vi "AB_Engine_InteropAssembly_Get_ProtoInfo.vi"(6 "2011CompatibilityMode":bool, 7 "Path":path, 8 "error in (no error)":errorcluster, 9 "destinations":refnum<class "AB_Destination.lvclass">[](array[class]), 11 "sourceItems":refnum<class "AB_Source.lvclass">[](array[class])) -> (0 "error out":errorcluster, 2 "ExportAssemblyLVClassinfo":T1[](array[typedef]), 3 "ExportAssemblyVIinfo":T3[](array[typedef]))   [LabVIEW 2020]
uses:
  <vilib>/AppBuilder/AB_Classes/Source/AB_Source.lvclass
  <vilib>/AppBuilder/AB_InteropAssembly_DistVI_Proto_Info.ctl
  <vilib>/AppBuilder/IOStatus.ctl
  <vilib>/AppBuilder/AB_Classes/Destination/AB_Destination.lvclass
  <vilib>/AppBuilder/AB_InteropAssembly_DistVI_Class_Info.ctl
  <vilib>/AppBuilder/AB_Classes/Source/ExportedAssemblyVI/AB_Source_Exported_Assembly_VI.lvclass
  <vilib>/Utility/lvfile.llb/NI_FileType.lvlib
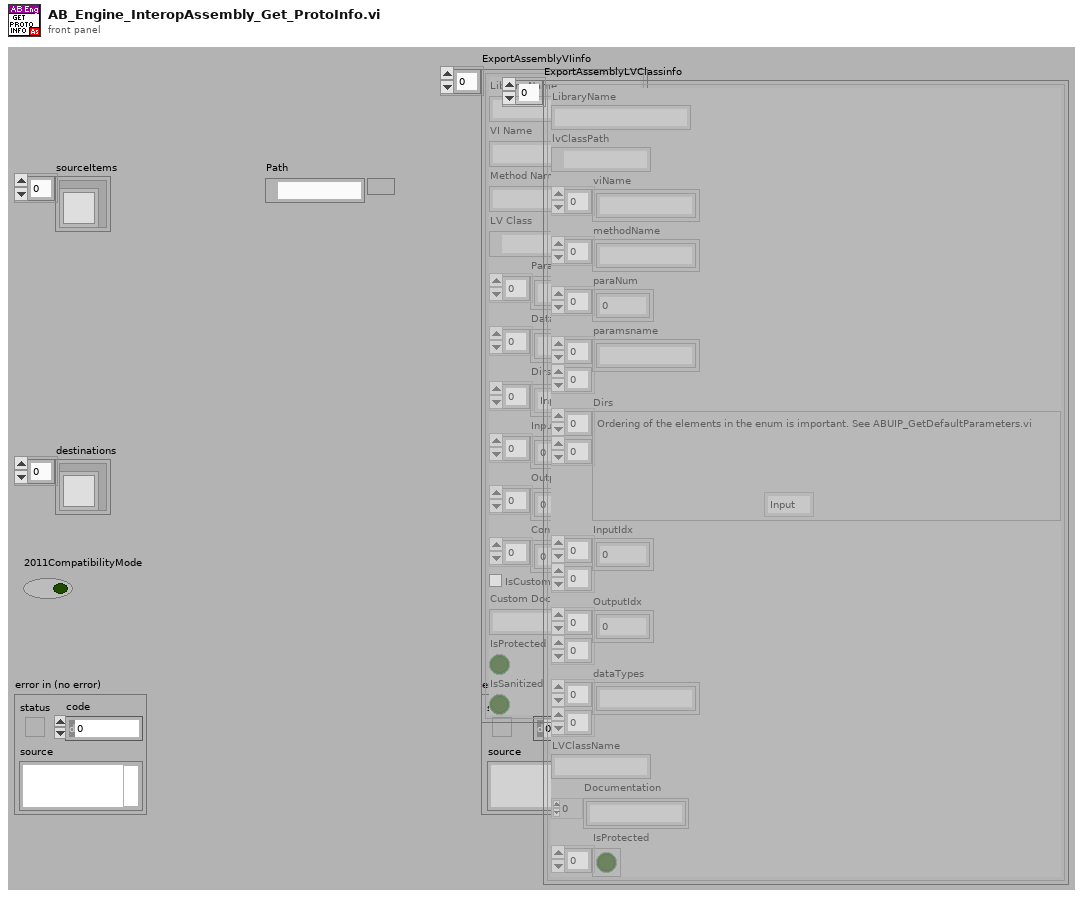
[diagram p1: front panel]
types:
  T1 = typedef "AB_InteropAssembly_DistVI_Class_Info.ctl" = cluster{"LibraryName":string, "lvClassPath":path, "viName":string[], "methodName":string[], "paraNum":i32[], "paramsname":string[][], "Dirs":T2[][], "InputIdx":i32[][], "OutputIdx":i32[][], "dataTypes":string[][], "LVClassName":string, "Documentation":string[], "IsProtected":bool[]}
  T2 = typedef "IOStatus.ctl" = enum16{"Input", "Output", "Input/Output", "InputDeleted", "OutputDeleted", "IODeleted", "ErrorClusterIn", "ErrorClusterOut"}
  T3 = typedef "AB_InteropAssembly_DistVI_Proto_Info.ctl" = cluster{"Library Name":string, "VI Name":string, "Method Name":string, "LV Class":path, "Param Names":string[], "Data Types":string[], "Dirs":T2[], "InputIdx":i32[], "OutputIdx":i32[], "ConNum":i8[], "IsCustomDocumentation":bool, "Custom Documentation":string, "IsProtected":bool, "IsSanitized":bool}
  T4 = cluster{"lvClassPath":path, "viName":string[], "methodName":string[], "paraNum":i32[], "paramsname":string[][], "Dirs":enum16{"in", "out", "in/out", "length"}[][], "InputIdx":i32[][], "OutputIdx":i32[][], "dataTypes":string[][], string}
  T5 = typedef "AB_Source.ctl" = cluster{"path":path, "itemID":string, "parentIndex":i32, "sourceInclusion":T6, "destinationIndex":i32, "properties":T7[], "newName":string, "lvfile":bool, "valid":bool, "eng_inBuild":bool, "eng_isNonVILink":bool, "Amalgamation":bool, "Amalgamation Piece":bool, "eng_delimitedName":string, "preventRename":bool}
  T6 = typedef "AB_Source_Inclusion.ctl" = enum16{"IncludeIfReferenced", "Include", "Exclude", "TopLevel"}
  T7 = typedef "AB_Source_Properties.ctl" = cluster{"sourcePropertyType":T8, "value":variant}
  T8 = typedef "AB_Source_Property_Type.ctl" = enum16{"Remove block diagram", "Remove front panel", "Password", "Window has title bar", "Show menu bar", "Show vertical scroll bar", "Show horizontal scroll bar", "Show toolbar", "Show Abort button", "Show fp when called", "Window behavior", "Allow user to close window", "Window run-time position", "Run when opened", "Allow debugging", "Auto error handling", "Generate guard code", "Use stack variables", "Expression folding", "Integer only", "Inline subVI"}
  T9 = typedef "AB_Destination.ctl" = cluster{"destName":string, "path":path, "libraryName":string, "preserveHierarchy":bool, "eng_inBuild":bool, "eng_libraryReference":refnum<vi>, "eng_restictAddToNewLibrary":bool}
  T10 = typedef "NI_FileType.lvlib/FT_FileTypes.ctl" = enum32{"Invalid file/path", "Unknown type", "Instrument", "Control", "Polymorphic VI", "Project", "Library", "LVClass", "XControl", "XNode", "CIN", "Run-time menu", "Palette menu", "LLB", "Shortcut", "Directory", "Class Private Data Control", "Statechart", "MathScript .m file", "Ladder Diagram", "LVLibp"}
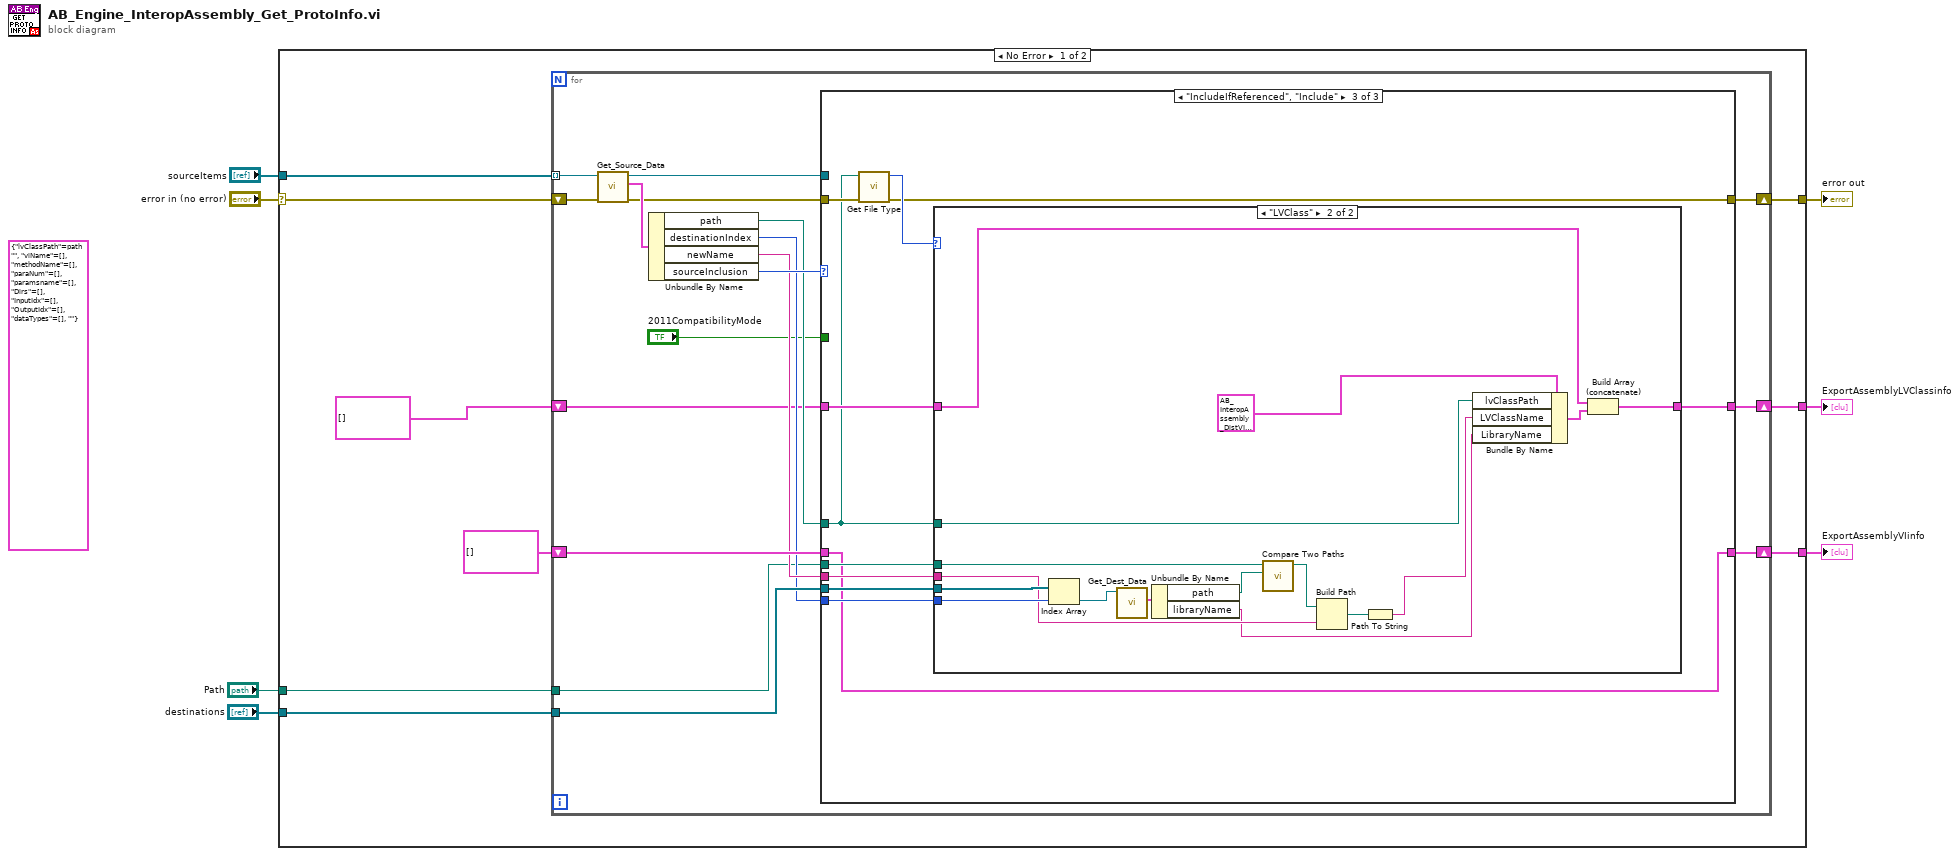
[diagram p0: block diagram]
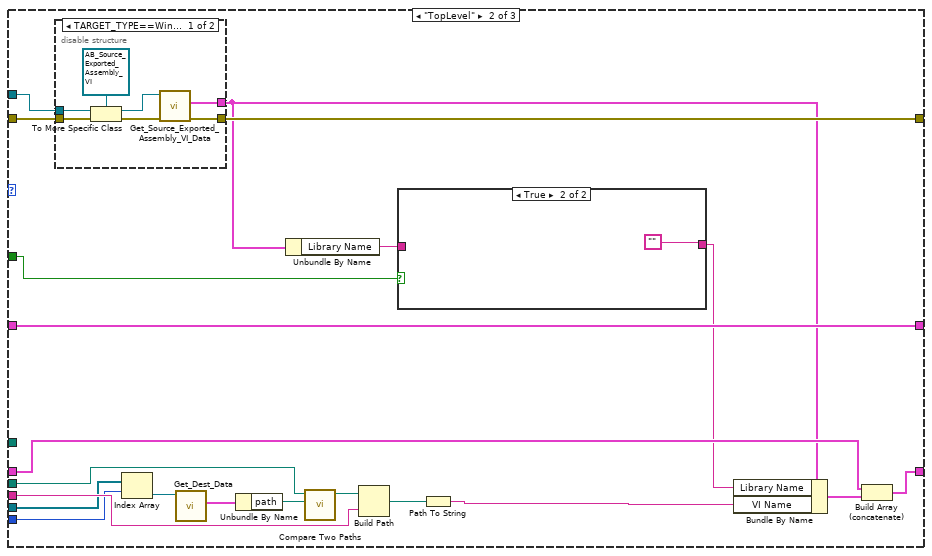
[diagram p3: hidden frame]
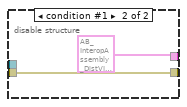
[diagram p5: hidden frame]
diagram:
  (unwired) T4 {"lvClassPath"=path "", "viName"=[], "methodName"=[], "paraNum"=[], "paramsname"=[], "Dirs"=[], "InputIdx"=[], "OutputIdx"=[], "dataTypes"=[], ""} ("ExportAssemblyVIinfo")
  n1 = case shown="No Error" "error in (no error)" {
    selector: "error in (no error)" -> [w15 w97]
    tunnel: "sourceItems" -> [w16 _]
    tunnel: [w14 _] -> w5
    tunnel: [w12 w97] -> w4
    tunnel: "destinations" -> [w11 _]
    tunnel: "Path" -> [w10 _]
    tunnel: [w8 _] -> w1
    frame No Error {
      n2 = for {
        tunnel: w16 -> [w32] mode=indexing
        shift-right: [w29] -> w12
        shift-left: w15 -> [w33]
        shift-right: [w31] -> w14
        shift-left: T3[] [] ("ExportAssemblyVIinfos") -> [w30]
        tunnel: w11 -> [w23]
        tunnel: w10 -> [w21]
        shift-right: [w18] -> w8
        shift-left: T1[] [] -> [w19]
        n3 = call <vilib>:"Get_Source_Data.vi"("error in (no error)"=w33, "Class in"=w32) -> ("error out"=w25:errorcluster, "data"=w28:T5, "Class out"=w26:refnum<class "AB_Source.lvclass">)  [unwired: 7 out]
        n4 = Unbundle By Name(w28) -> ("path"=w20:path, "destinationIndex"=w22:i32, "newName"=w24:string, "sourceInclusion"=w27:T6)
        n5 = case shown="\"IncludeIfReferenced\", \"Include\"" w27 {
          tunnel: w26 -> [_ w55 _]
          tunnel: w25 -> [w35 w54 w73]
          tunnel: [w36 w57 w74] -> w31
          tunnel: w30 -> [w36 w56 w74]
          tunnel: [w35 w53 w72] -> w29
          tunnel: w24 -> [_ w52 w77]
          tunnel: w23 -> [_ w49 w78]
          tunnel: w22 -> [_ w48 w79]
          tunnel: w21 -> [_ w47 w76]
          tunnel: w20 -> [_ _ w69]
          tunnel: w19 -> [w34 w46 w71]
          tunnel: [w34 w46 w70] -> w18
          tunnel: "2011CompatibilityMode" -> [_ w44 _]
          frame Default {
          }
          frame "TopLevel" {
            n6 = disable-structure shown="TARGET_TYPE==Windows" {
              disable-tunnel: w55 -> [w64 _]
              disable-tunnel: w54 -> [w63 w68]
              disable-tunnel: [w62 w68] -> w53
              disable-tunnel: [w61 T3 {"Library Name"="", "VI Name"="", "Method Name"="", "LV Class"=path "", "Param Names"=[], "Data Types"=[], "Dirs"=[], "InputIdx"=[], "OutputIdx"=[], "ConNum"=[], "IsCustomDocumentation"=FALSE, "Custom Documentation"="", "IsProtected"=FALSE, "IsSanitized"=FALSE} ("ExportAssemblyVIinfo")] -> w45
              frame condition #0 (active) {
                n7 = To More Specific Class(target class=refnum<class "AB_Source_Exported_Assembly_VI.lvclass"> refnum ("AB_Source_Exported_Assembly_VI.lvclass"), reference=w64, error in=w63) -> (specific class reference=w60:refnum<class "AB_Source_Exported_Assembly_VI.lvclass">, error out=w65:errorcluster)
                n8 = call <vilib>:"Get_Source_Exported_Assembly_VI_Data.vi"("error in (no error)"=w65, "AB_Source_Exported_Assembly_VI.lvclass in"=w60) -> ("error out"=w62:errorcluster, "ExportAssemblyVIinfo"=w61:T3)  [unwired: 8 out]
              }
              frame condition #1 {
              }
            }
            n9 = Index Array(array=w49, index=w48) -> (element=w41:refnum<class "AB_Destination.lvclass">)
            n10 = call <vilib>:"Get_Dest_Data.vi"("Class in"=w41) -> ("destName"=w40:T9)  [unwired: 1 in, 9 out]
            n11 = Unbundle By Name(w40) -> ("path"=w39:path)
            n12 = Unbundle By Name(w45) -> ("Library Name"=w43:string)
            n13 = call <vilib>:"Compare Two Paths.vi"("Path 2"=w39, "Path 1"=w47) -> ("Relative Path from 1 to 2"=w38:path)  [unwired: 1 in, 8 out]
            n14 = Build Path(base path=w38, name or relative path=w52) -> (appended path=w37:path)
            n15 = case shown="True" w44 {
              tunnel: w43 -> [w58 _]
              tunnel: [w58 ""] -> w42
              frame False {
              }
              frame True {
              }
            }
            n16 = Path To String(path=w37) -> (string=w51:string)
            n17 = Bundle By Name(cluster=w45, "Library Name"=w42, "VI Name"=w51) -> (w50:T3)
            n18 = Build Array (concatenate)(w56, w50) -> (w57:T3[])
          }
          frame "IncludeIfReferenced", "Include" {
            n19 = call <vilib>:"Get File Type.vi"("error in (no error)"=w73, "path"=w69) -> ("error out"=w72:errorcluster, "file type"=w75:T10)  [unwired: 7 in, 1 out]
            n20 = case shown="\"LVClass\"" w75 {
              tunnel: w79 -> [_ w96]
              tunnel: w78 -> [_ w95]
              tunnel: w77 -> [_ w94]
              tunnel: w76 -> [_ w93]
              tunnel: w71 -> [w80 w92]
              tunnel: [w80 w91] -> w70
              tunnel: w69 -> [_ w88]
              frame "Invalid file/path", Default {
              }
              frame "LVClass" {
                n21 = Index Array(array=w95, index=w96) -> (element=w85:refnum<class "AB_Destination.lvclass">)
                n22 = call <vilib>:"Get_Dest_Data.vi"("Class in"=w85) -> ("destName"=w84:T9)  [unwired: 1 in, 9 out]
                n23 = Unbundle By Name(w84) -> ("path"=w83:path, "libraryName"=w87:string)
                n24 = call <vilib>:"Compare Two Paths.vi"("Path 2"=w83, "Path 1"=w93) -> ("Relative Path from 1 to 2"=w82:path)  [unwired: 1 in, 8 out]
                n25 = Build Path(base path=w82, name or relative path=w94) -> (appended path=w81:path)
                n26 = Path To String(path=w81) -> (string=w90:string)
                n27 = Bundle By Name(cluster=T1 {"LibraryName"="", "lvClassPath"=path "", "viName"=[], "methodName"=[], "paraNum"=[], "paramsname"=[], "Dirs"=[], "InputIdx"=[], "OutputIdx"=[], "dataTypes"=[], "LVClassName"="", "Documentation"=[], "IsProtected"=[]} ("ExportAssemblyVIinfo"), "lvClassPath"=w88, "LVClassName"=w90, "LibraryName"=w87) -> (w89:T1)
                n28 = Build Array (concatenate)(w92, w89) -> (w91:T1[])
              }
            }
          }
        }
      }
    }
    frame Error {
    }
  }
  "error out" <- w4
  "ExportAssemblyVIinfo" <- w5
  "ExportAssemblyLVClassinfo" <- w1
